vi "BRig_arrTrig_CueAudio_R.vi"() -> (2 "output_CueAudio_R":i32)   [LabVIEW 2014]
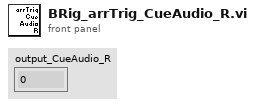
[diagram p1: front panel]
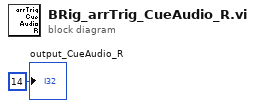
[diagram p0: block diagram]
diagram:
  "output_CueAudio_R" <- 14
